vi "NewIndependentGen.vi"() -> ()   [LabVIEW 2020]
uses:
  Generator_States.ctl
  <instrlib>/_niInstr/Basic Elements/v1/FPGA/niInstr Basic Elements v1 FPGA.lvlib
panel:
  in  "Send vi Trig":bool
  out "Gain":dbl
  out "Offset Factor":dbl
  out "Amplitudes":dbl[](array[numeric]) format="%.2f"
  out "Sampling Frequency (Hz)":u64
  out "Waves per Pixel":u32
  in  "Generator  Port":refnum<k15>
  out "Actual Sample Rate":dbl format="%#_6p"
  in  "Use Default Wave Settings":bool caption="Checkbox"
  in  "Start Gen":bool
  in  "stop Gen":bool
  out "Generator On":bool
  out "Input Waveform":dbl[](graph)
  in  "Ext/nViTrig":bool=TRUE
  in  "Stop Generator \nApplication":bool
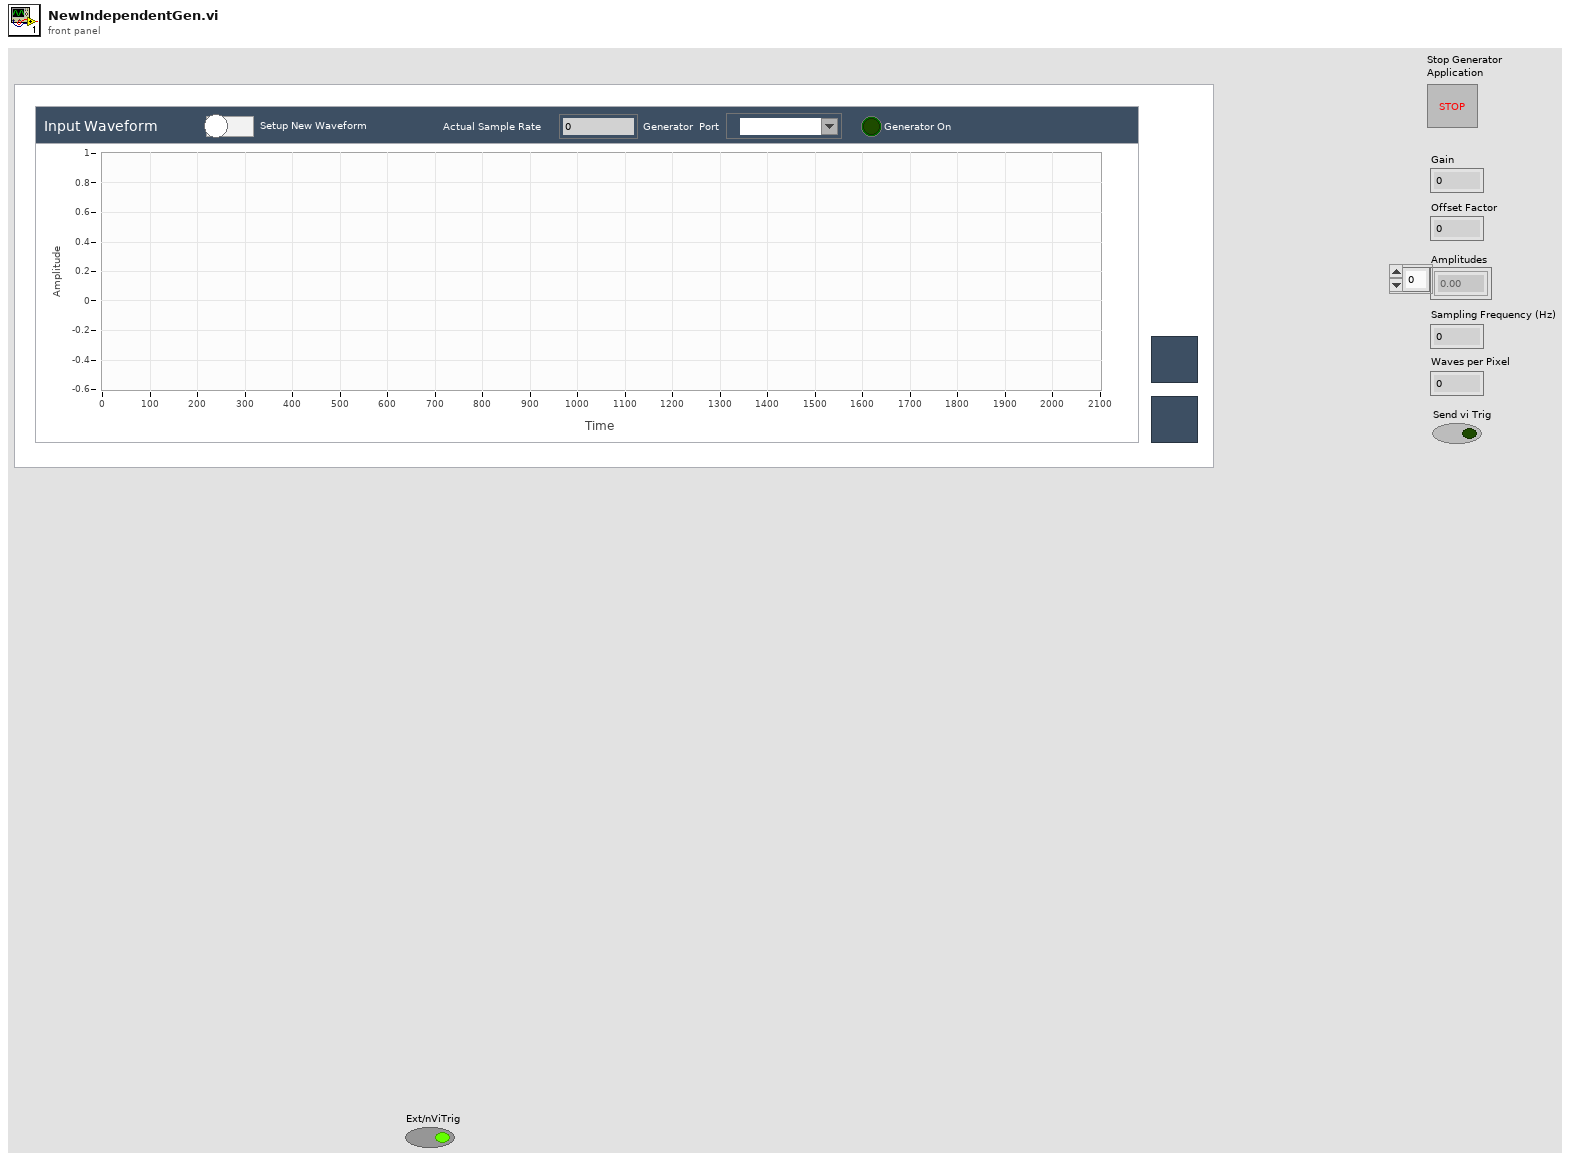
[diagram p1: front panel]
types:
  T1 = typedef "Generator_States.ctl" = enum16{"Idle", "GenerateWaveArray", "InitGen", "SendVITrig", "CloseGen", "CloseApp"}
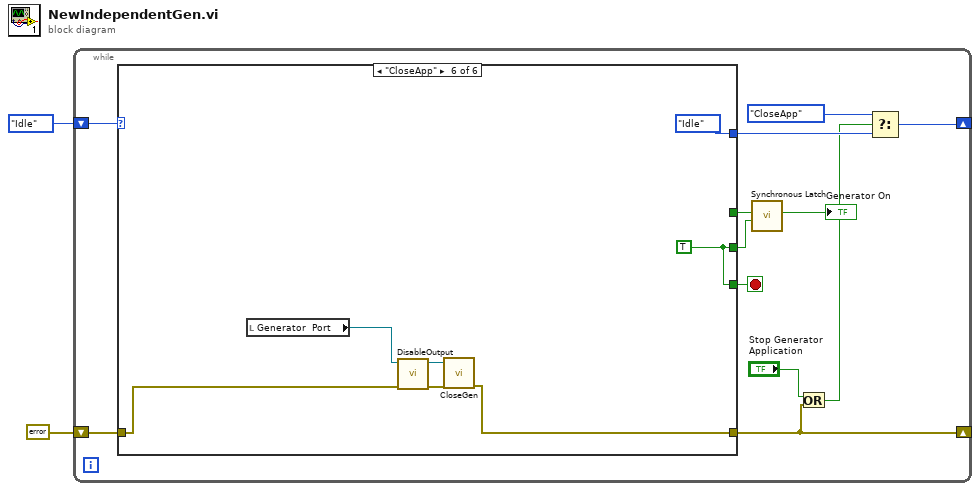
[diagram p0: block diagram]
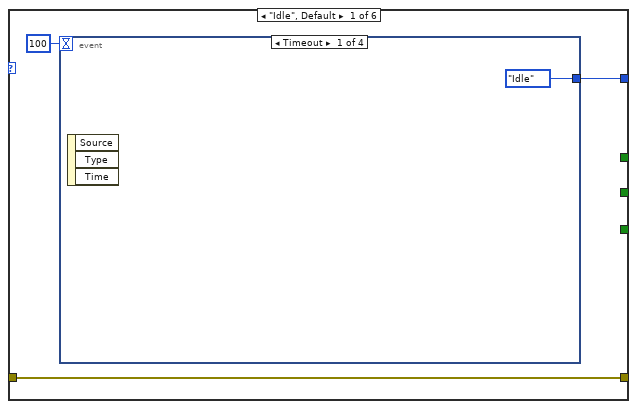
[diagram p2: hidden frame]
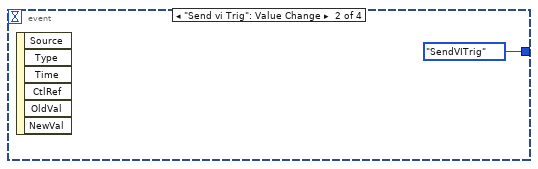
[diagram p3: hidden frame]
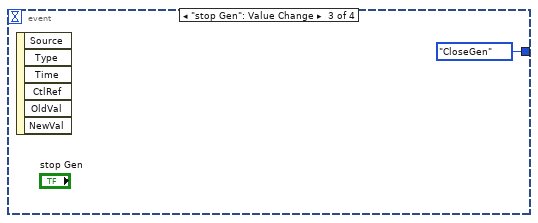
[diagram p4: hidden frame]
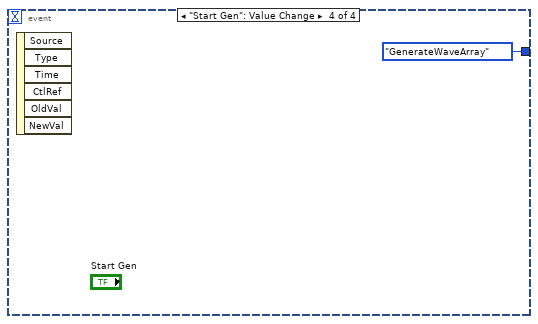
[diagram p5: hidden frame]
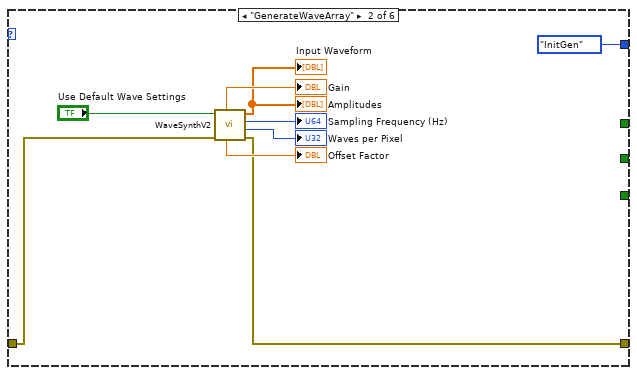
[diagram p6: hidden frame]
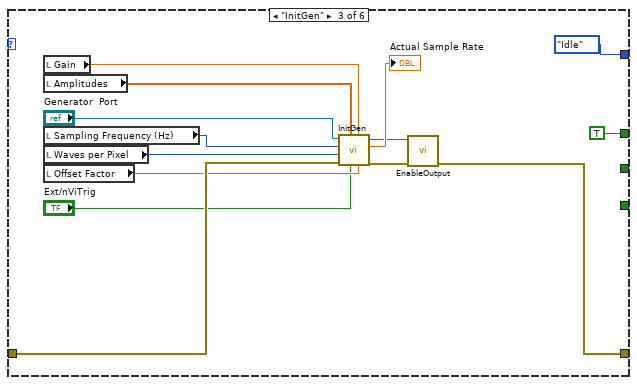
[diagram p7: hidden frame]
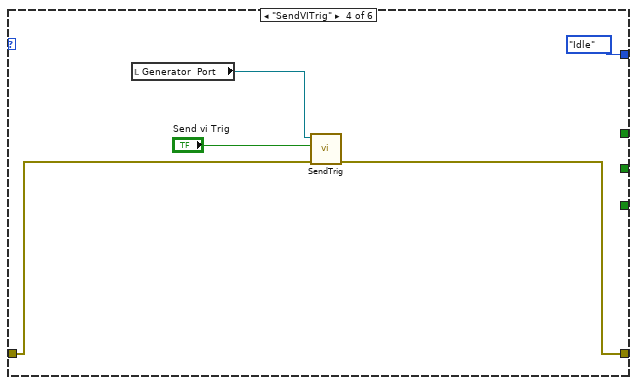
[diagram p8: hidden frame]
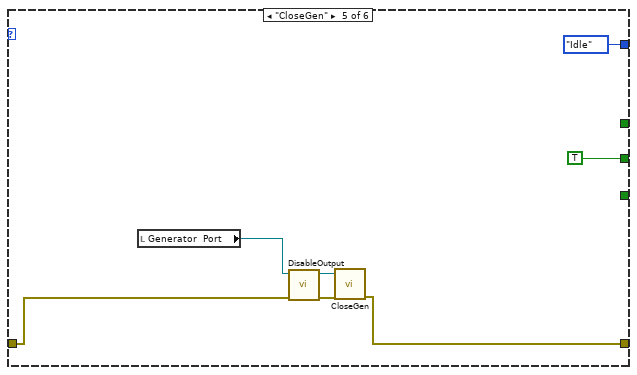
[diagram p9: hidden frame]
diagram:
  n1 = while {
    shift-right: [w11] -> _
    shift-left: Generator_States."Idle" -> [w14]
    shift-right: [w12] -> _
    shift-left: errorcluster {"status"=FALSE, "code"=0, "source"=""} ("error in") -> [w13]
    stop <- w3 stop-if-true
    n2 = case shown="\"CloseApp\"" w14 {
      tunnel: [w16 Generator_States."InitGen" Generator_States."Idle" Generator_States."Idle" Generator_States."Idle" Generator_States."Idle"] -> w10
      tunnel: w13 -> [w15 w30 w43 w49 w54 w61]
      tunnel: [w15 w24 w34 w48 w53 w60] -> w12
      tunnel: [_ _ TRUE ("Ext/nViTrig") _ _ _] -> w8
      tunnel: [_ _ _ _ TRUE ("x .or. y?") w57] -> w7
      tunnel: [_ _ _ _ _ w57] -> w3
      frame "Idle", Default {
        n3 = event shown="[0] Timeout" {
          selector: _ -> [_ _ _ _]
          dyn-events: _ -> [_ _ _ _]
          timeout: 100 -> [_ _ _ _]
          tunnel: [Generator_States."Idle" Generator_States."SendVITrig" Generator_States."CloseGen" Generator_States."GenerateWaveArray"] -> w16
          event Timeout {
            n4 = event-data() -> ()  [unwired: 1 in, 3 out]
          }
          event "Send vi Trig": Value Change {
            n5 = event-data() -> ()  [unwired: 1 in, 6 out]
          }
          event "stop Gen": Value Change {
            n6 = event-data() -> ()  [unwired: 1 in, 6 out]
          }
          event "Start Gen": Value Change {
            n7 = event-data() -> ()  [unwired: 1 in, 6 out]
          }
        }
      }
      frame "GenerateWaveArray" {
        n8 = call "WaveSynthV2.vi"("error in"=w30, "Default Wave"="Use Default Wave Settings") -> ("error out"=w24:errorcluster, "Waves per Pixel"=→"Waves per Pixel":u32, "Sampling Frequency (Hz)"=→"Sampling Frequency (Hz)":u64, "Amplitudes"=→"Amplitudes" →"Input Waveform":dbl[], "Offset Factor"=→"Offset Factor":dbl, "Gain"=→"Gain":dbl)  [unwired: 2 in]
      }
      frame "InitGen" {
        n9 = local read "Gain"() -> (w38:dbl)
        n10 = local read "Amplitudes"() -> (w39:dbl[])
        n11 = local read "Sampling Frequency (Hz)"() -> (w41:u64)
        n12 = local read "Waves per Pixel"() -> (w40:u32)
        n13 = local read "Offset Factor"() -> (w37:dbl)
        n14 = call "InitGen.vi"("Offset"=w37, "Gain"=w38, "Ext/nViTrig"="Ext/nViTrig", "Waveform Data Array"=w39, "error in (no error)"=w43, "Wave Per Pixel"=w40, "Sample Rate (Samp/s)"=w41, "FGEN Resource Name"="Generator  Port") -> ("error out"=w35:errorcluster, "Actual Sample Rate"=→"Actual Sample Rate":dbl, "reference out"=w33:refnum<k15>)  [unwired: 1 in]
        n15 = call "EnableOutput.vi"("error in (no error)"=w35, "FGEN Resource Name"=w33) -> ("error out"=w34:errorcluster)  [unwired: 8 in, 1 out]
      }
      frame "SendVITrig" {
        n16 = local read "Generator  Port"() -> (w45:refnum<k15>)
        n17 = call "SendTrig.vi"("error in (no error)"=w49, "Send vi Trig"="Send vi Trig", "Instrument Handle"=w45) -> ("error out"=w48:errorcluster)  [unwired: 7 in, 1 out]
      }
      frame "CloseGen" {
        n18 = local read "Generator  Port"() -> (w52:refnum<k15>)
        n19 = call "DisableOutput.vi"("error in (no error)"=w54, "FGEN Resource Name"=w52) -> ("error out"=w56:errorcluster, "Instrument Handle Out"=w55:refnum<k15>)  [unwired: 8 in]
        n20 = call "CloseGen.vi"("error in (no error)"=w56, "Instrument Handle"=w55) -> ("error out"=w53:errorcluster)  [unwired: 9 in]
      }
      frame "CloseApp" {
        w57 = TRUE ("x .or. y?")
        n21 = local read "Generator  Port"() -> (w59:refnum<k15>)
        n22 = call "DisableOutput.vi"("error in (no error)"=w61, "FGEN Resource Name"=w59) -> ("error out"=w63:errorcluster, "Instrument Handle Out"=w62:refnum<k15>)  [unwired: 8 in]
        n23 = call "CloseGen.vi"("error in (no error)"=w63, "Instrument Handle"=w62) -> ("error out"=w60:errorcluster)  [unwired: 9 in]
      }
    }
    n24 = call <instrlib>:"Synchronous Latch.vi"("clear"=w7, "set"=w8) -> ("out"=→"Generator On":bool)  [unwired: 9 in]
    n25 = Or(x="Stop Generator \nApplication", y=w12) -> (x .or. y?=w4:bool)
    n26 = Select(t=Generator_States."CloseApp", s=w4, f=w10) -> (s? t:f=w11:T1)
  }
